vi "FPGA Configure FIFO By Name.vi"(8 "error in (no error)":errorcluster, 9 "Depth":u64, 10 "FIFO":string, 11 "FPGA Session In":refnum<class "FPGA Interface Base.lvclass">) -> (0 "error out":errorcluster, 3 "FPGA Session Out":refnum<class "FPGA Interface Base.lvclass">)   [LabVIEW 2010, in "FPGA Interface Base.lvclass"]
doc: "Specifies the depth of the host memory part of the DMA FIFO. This method is optional."
uses:
  <userlib>/_FPGA Interface Advanced Tools/FPGA Interface Base/FPGA Interface Base.lvclass
  <userlib>/_FPGA Interface Advanced Tools/FPGA Interface Base/FPGA Interface Base.lvclass/FPGA Interface Base.ctl
  <vilib>/Utility/error.llb/Error Cluster From Error Code.vi
  <userlib>/_FPGA Interface Advanced Tools/FPGA Interface Base/Accessors/FPGA Read Session.vi
  <userlib>/_FPGA Interface Advanced Tools/FPGA Interface Wrapper/FPGA Interface Wrapper.lvlib
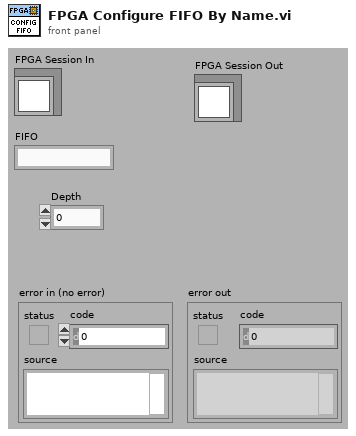
[diagram p1: front panel]
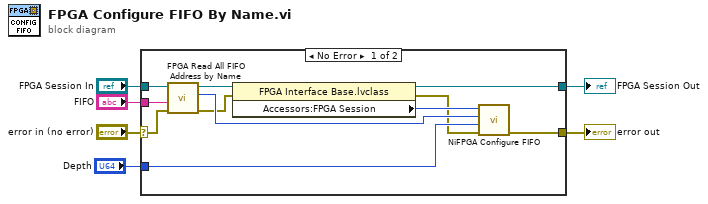
[diagram p0: block diagram]
diagram:
  n1 = case shown="No Error" "error in (no error)" {
    selector: "error in (no error)" -> [w15 w19]
    tunnel: [w7 w19] -> w3
    tunnel: [w8 w18] -> w5
    tunnel: "FPGA Session In" -> [w16 w18]
    tunnel: "FIFO" -> [w14 _]
    tunnel: "Depth" -> [w17 _]
    frame No Error {
      n2 = call <userlib>:"FPGA Read All FIFO Address by Name.vi"("error in (no error)"=w15, "Name"=w14, "FPGA Interface Base in"=w16) -> ("error out"=w11:errorcluster, "Address"=w13:u32, "FPGA Interface Base out"=w12:refnum<class "FPGA Interface Base.lvclass">)  [unwired: 5 in, 1 out]
      n3 = property class="FPGA Interface Base.lvclass"(reference=w12, error in=w11) -> (reference out=w8:refnum<class "FPGA Interface Base.lvclass">, error out=w9:errorcluster, "Accessors:FPGA Session"=w10:u32)
      n4 = call <userlib>:"NiFPGA Configure FIFO.vi"("error in (no error)"=w9, "Depth"=w17, "FIFO"=w13, "Session"=w10) -> ("error out"=w7:errorcluster)  [unwired: 6 in, 1 out]
    }
    frame Error {
    }
  }
  "error out" <- w3
  "FPGA Session Out" <- w5
